vi "jettl Msg Create Event.vi"(9 "Event":refnum<class "Event.lvclass">, 10 "Self Event Alias":string) -> (2 "Msg Strategy":refnum<class "Msg Strategy.lvclass">)   [LabVIEW 2021, in "jettl Msg Create Event.lvlib"]
uses:
  jettl Msg Create Event.lvlib
  jettl/Event/Event.lvclass
  jettl/Msg Strategy/Msg Strategy.lvclass
  Create Event Msg Strategy/Create Event Msg Strategy.lvclass
  C:/git/jettl/src/jettl/Msg Strategy/Msg Strategy.lvclass
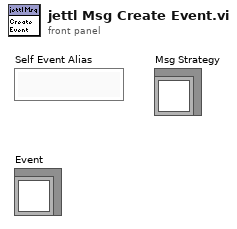
[diagram p1: front panel]
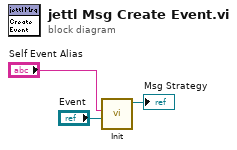
[diagram p0: block diagram]
diagram:
  n1 = call "Init.vi"("Event"="Event", "Self Event Alias"="Self Event Alias") -> ("Create Event Msg Strategy out"=→"Msg Strategy":refnum<class "Create Event Msg Strategy.lvclass">)  [unwired: 9 in]
